vi "Create MQTT Client.vi"(5 "Client in":refnum<class "Client.lvclass">, 8 "error in (no error)":errorcluster, 11 "ID (empty:generate new)":string) -> (0 "error out":errorcluster, 3 "Client out":refnum<class "Client.lvclass">)   [LabVIEW 2013, in "MQTT Server.lvlib" / "Client.lvclass"]
uses:
  Client.lvclass
  Client.lvclass/Client.ctl
  Control Packets/ControlPacket/ControlPacket.lvclass
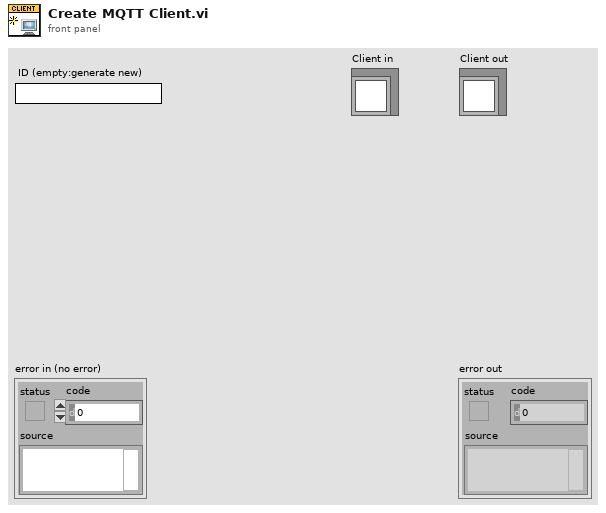
[diagram p1: front panel]
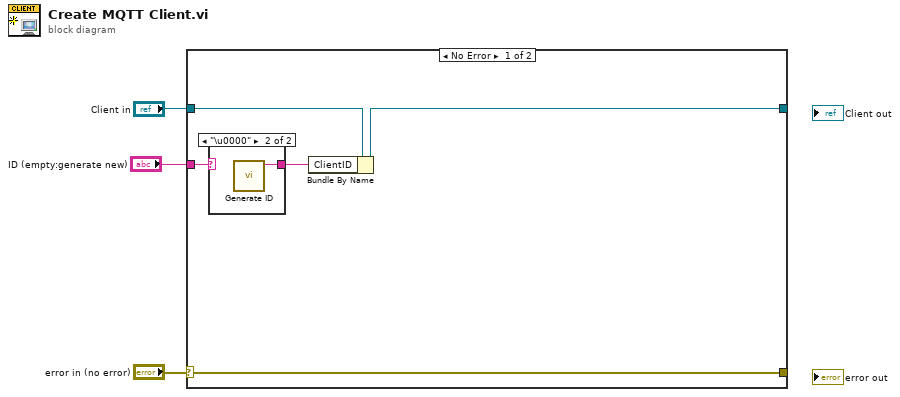
[diagram p0: block diagram]
diagram:
  n1 = case shown="No Error" "error in (no error)" {
    selector: "error in (no error)" -> [w8 w12]
    tunnel: [w8 w12] -> _
    tunnel: [w6 w11] -> _
    tunnel: "Client in" -> [w7 w11]
    tunnel: "ID (empty:generate new)" -> [w5 _]
    frame No Error {
      n2 = case shown="\"\"" w5 {
        selector: w5 -> [w9 _]
        tunnel: [w9 w10] -> w4
        frame Default {
        }
        frame "\u0000" {
          n3 = call "Generate ID.vi"() -> ("ID"=w10:string)  [unwired: 11 in]
        }
      }
      n4 = Bundle By Name(cluster=w7, "ClientID"=w4) -> (w6:refnum<class "Client.lvclass">)
    }
    frame Error {
    }
  }
